vi "Comm Error Check2 (SubVI).vi"(0 "Number of Arguments":i32, 1 "Reply string array":string[](array[string]), 2 "error in (no error)":errorcluster, 3 "Reply string":string, 4 "Error Source String 2":string, 5 "Error Source String 1":string) -> ()   [LabVIEW 2020]
doc: "Checks instrument reply message (must be wired to the \"result string\" input terminal) and looking for \"ERROR#\" string. If found displays dialog box with message string wired to the \"Error Source String\" terminal. This SubVI will block program execution if instrument replies with error message. If your application should not be interrupted do not use this SubVI. In addition, it checks number of the element in the array wired to the \"Reply String Array\" terminal and compares it with \"Number of Element\" value. If not equal provide additional message (the text of the message must be wired to the \"Error Source #2\" terminal) in the dialog box. This SubVI can be used to verify coma delimited string reply message (must be converted in to array of strings)."
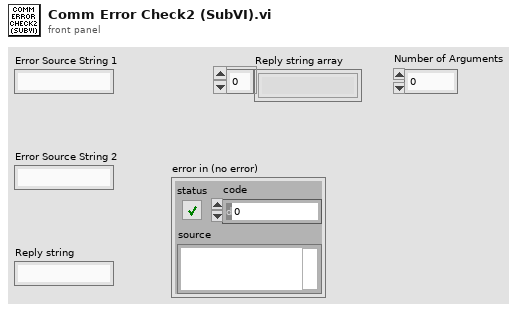
[diagram p1: front panel]
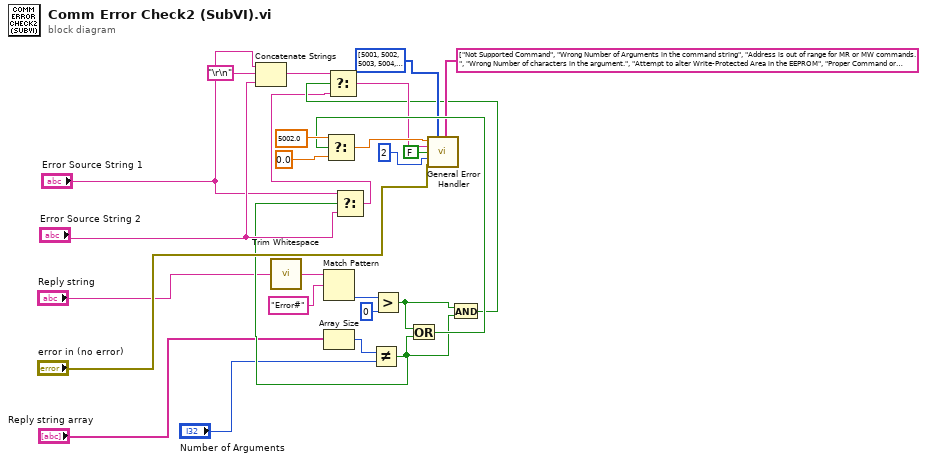
[diagram p0: block diagram]
diagram:
  n1 = Concatenate Strings("Error Source String 1", "\r\n", "Error Source String 2") -> (w10:string)
  n2 = call <vilib>:"Trim Whitespace.vi"("string"="Reply string") -> ("trimmed string"=w7:string)  [unwired: 1 in]
  n3 = Match Pattern(string=w7, regular expression="Error#") -> (offset past match=w4:i32)  [unwired: 1 in, 3 out]
  n4 = Array Size(array="Reply string array") -> (size(s)=w6:i32)
  n5 = Not Equal?(x=w6, y="Number of Arguments") -> (x != y?=w12:bool)
  n6 = Select(t="Error Source String 1", s=w12, f="Error Source String 2") -> (s? t:f=w11:string)
  n7 = Greater?(x=w4, y=0) -> (0:w13:bool)
  n8 = Or(x=w13, y=w12) -> (x .or. y?=w23:bool)
  n9 = Select(t=5002.0, s=w23, f=0.0) -> (s? t:f=w25:dbl)
  n10 = And(x=w13, y=w12) -> (x .and. y?=w14:bool)
  n11 = Select(t=w10, s=w14, f=w11) -> (s? t:f=w19:string)
  n12 = call <vilib>:"General Error Handler.vi"("[error code] (0)"=w25, "[user-defined codes]"=i32[] [5001, 5002, 5003, 5004, 5005, 5006, 5007, 5008, 5009], "[user-defined descriptions]"=string[] ["Not Supported Command", "Wrong Number of Arguments in the command string", "Address is out of range for MR or MW commands.", "Wrong Number of characters in the argument.", "Attempt to alter Write-Protected Area in the EEPROM", "Proper Command or Argument not found", "Wrong value of the Argument in the command string.", "Wrong value of the Argument", "Manufacturer-specific information EE access KEY (wrong key or key is disabled.", "No Description evailable for this Error code."], "[error source] (\" \")"=w19, "search ni.com link visible?(T)"=FALSE, "type of dialog (OK msg:1)"=2, "error in (no error)"="error in (no error)") -> ()  [unwired: 4 in, 5 out]
